vi "RT Driver VI.vi"(6 "Device Clock":string, 9 "Device Inputs FIFO":refnum<k33>, 10 "Device Outputs FIFO":refnum<k33>, 11 "Device Reference":T1 format="%.0x") -> ()   [LabVIEW 2018, in "CAN Gateway Engine.lvlib"]
uses:
  CAN Gateway Engine.lvlib
  <vilib>/NI Veristand/Custom Device API/Custom Device Item Ref.ctl
  <vilib>/Platform/TimedLoop/XDataNode/timing_clust.ctl
  <vilib>/Platform/TimedLoop/XDataNode/nitl_modes.ctl
  <vilib>/Platform/TimedLoop/XDataNode/wakeup.ctl
  <vilib>/platform/TimedLoop/XDataNode/XDataNode.xnode
  <vilib>/Platform/TimedLoop/XDataNode/XDNodeRunTimeDep.lvlib
  <vilib>/NI Veristand/Custom Device API/Custom Device API.lvlib
panel:
  in  "Initialization Status Notifier":refnum<notifier>
  in  "Status Notifier":refnum<notifier>
  # "Custom Device Template\nv1.0"
  # "Use this template as a starting point for creating a custom device code module. The input controls shown here are specially named controls that the system will use to provide the device loop with data. The controls are not required for the device loop to run. For instance, if the device doesn't produce any output data, then you don't need the Device Outputs FIFO control. If you do use these controls, however, they need to have these exact names to be functional."
  # "The optional status notifier element is used to notify the RT engine of the last state of the custom device, and to indicate the device has completed execution. If this control is not used, a default No Error value is returned to the system when the device finishes execution.\n\nNote: This error state is not checked until the system shuts down. Use an output status channel to send more immediate status values to the system."
  # "This optional input can be used to send the VeriStand Engine the final status of the custom device initalization process. If this control exists on the custom device front panel, the VeriStand Engine will wait for a status update before starting up. If the custom device reports an error, that will abort the execution of the current configuration in the VeriStand Engine.\n\nThis control can be deleted if the custom device does not need to send the initialization status update."
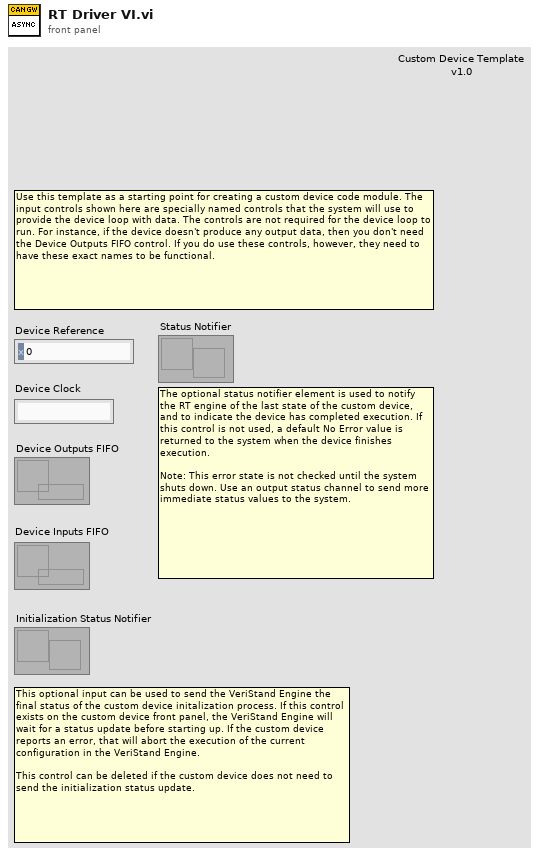
[diagram p1: front panel]
types:
  T1 = typedef "Custom Device API.lvlib/Custom Device Item Ref.ctl" = u64
  T2 = typedef "CAN Gateway Engine.lvlib/Runtime engine Data.ctl" = cluster{"Device Outputs FIFO":refnum<k33>, "Device Inputs FIFO":refnum<k33>, "CD In Size":i32, "CD Out Size":i32, "CD In Buf":dbl[], "CD Out Buf":dbl[], "Event Registration Refnum out":T3, "Specified Channel Ref List In":T1[], "Specified Channel Ref List Out":T1[], "Compiled Data":T4, "Read /write Sessions":cluster{"Network Read Session":refnum<k21>, "Network Write Session":refnum<k21>, "DUT Read Session":refnum<k21>, "DUT Write Session":refnum<k21>}}
  T3 = typedef "Custom Device API.lvlib/Custom Device Engine Event Ref.ctl" = refnum<event-registration>
  T4 = typedef "CAN Gateway Shared.lvlib/Compiled Data.ctl" = cluster{"HW Info Network Port":cluster{"CAN Port":string, "Baudrate":u64}, "HW Info DUT Port":cluster{"CAN Port":string, "Baudrate":u64}, "Corruption Info Network_DUT":T5, "Corruption Info DUT_Network":T5}
  T5 = typedef "CAN Gateway Shared.lvlib/Corruption Info.ctl" = cluster{"Corrupt IDs Array":u32[], "Frame Infos Array":T6[]}
  T6 = typedef "CAN Gateway Shared.lvlib/Frame.ctl" = cluster{"Disable Frame Channel Index":i32, "Has  CRC?":bool, "CRC start Bit":u32, "DLC corruption Channel Index":i32, "DLC Length  Corruption Index":i32, "CRC Index":i32, "Conversion Session":refnum<k21>, "CRC Signal":refnum<k21>, "Data Signal Array":T7[]}
  T7 = typedef "CAN Gateway Shared.lvlib/Signal_Data_Trigger.ctl" = cluster{"XNET Signal":refnum<k21>, "Data Idx":u32, "Trigger Idx":u32}
  T8 = typedef "XDNodeRunTimeDep.lvlib/timing_clust.ctl" = cluster{"Expected End [f-1]":u64, "Actual End [f-1]":u64, "Finished Late? [f-1]":bool, "Expected End [i-1]":u64, "Actual End [i-1]":u64, "Finished Late? [i-1]":bool, "Expected Start [i]":u64, "Actual Start [i]":u64, "Expected Start [f]":u64, "Actual Start [f]":u64, "Source Name":string, "Structure Name":string, "Period":i64, "Deadline":i64, "Offset":i64, "Start":i64, "Priority":i32, "Timeout":i32, "Mode":T9, "Wakeup Reason":T10, "Error":errorcluster, "Source Type":string, "Secondary Source Type":string, "Global End Time":u64, "Global Start Time":u64, "Frame Duration":u64, "Iteration Duration":u64, "Assigned CPU":i32, "I/O Scan Engine Mode":u32}
  T9 = typedef "XDNodeRunTimeDep.lvlib/nitl_modes.ctl" = enum32{"No Change", "Process missed periods, maintain original phase", "Discard missed periods, maintain original phase", "Process missed periods, ignore original phase", "Discard missed periods, ignore original phase"}
  T10 = typedef "XDNodeRunTimeDep.lvlib/wakeup.ctl" = enum32{"Normal", "Aborted", "Asynchronous wakeup", "Timing source error", "Timed loop error", "Timeout"}
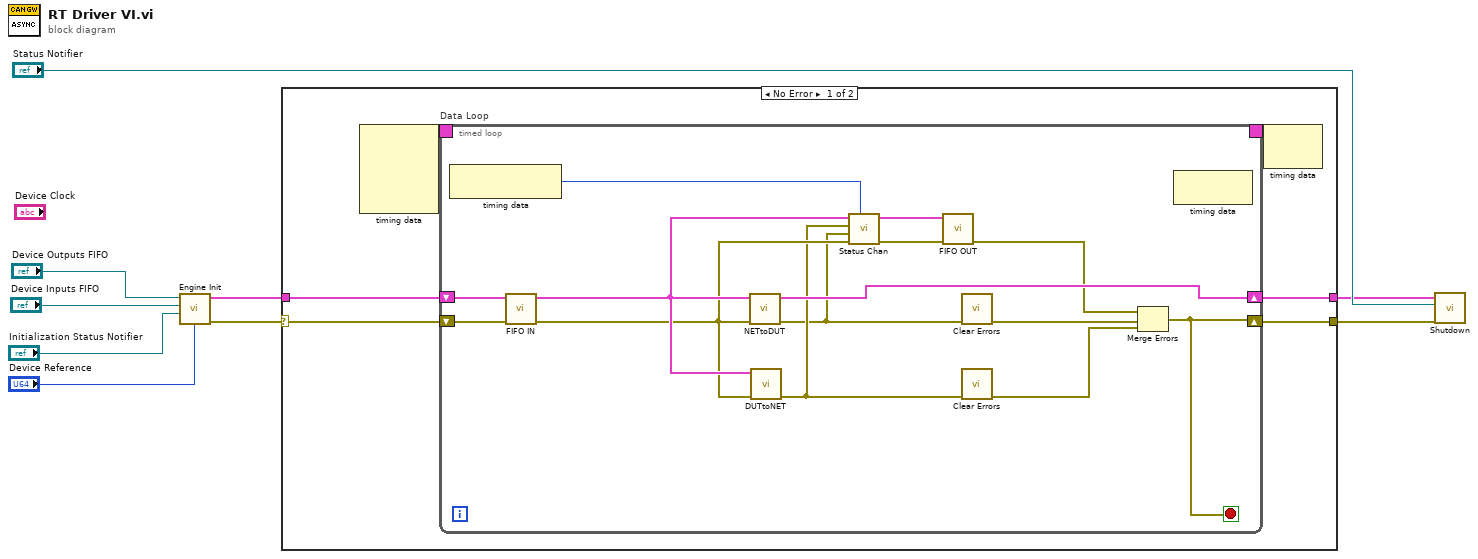
[diagram p0: block diagram]
diagram:
  n1 = call "Engine Init.vi"("Device Reference"="Device Reference", "Notifier in"="Initialization Status Notifier", "Device Inputs FIFO"="Device Inputs FIFO", "Device Outputs FIFO"="Device Outputs FIFO") -> ("error out"=w8:errorcluster, "Engine Run-Time Data Cluster"=w9:T2)  [unwired: 6 in]
  n2 = case shown="No Error" w8 {
    selector: w8 -> [w14 w36]
    tunnel: w9 -> [w11 w35]
    tunnel: [w15 w36] -> w3
    tunnel: [w10 w35] -> w1
    frame No Error {
      n3 = node-c288() -> (w13:T8)  [unwired: 4 in]
      n4 = timed-loop "Data Loop" {
        shift-right: [w23] -> w15
        shift-left: w14 -> [w29]
        shift-right: [w20] -> w10
        shift-left: w11 -> [w28]
        timing: w13 -> [_]
        timing-out: [_] -> w12
        stop <- w23 stop-if-true
        n5 = node-c288() -> (w18:i64)  [unwired: 1 in]
        n6 = call "FIFO IN.vi"("error in (no error)"=w29, "Engine Run-Time Data Cluster In"=w28) -> ("error out"=w26:errorcluster, "Engine Run-Time Data Cluster Out"=w27:T2)  [unwired: 8 in]
        n7 = call "NETtoDUT.vi"("error in (no error)"=w26, "Engine Run-Time Data Cluster In"=w27) -> ("error out"=w16:errorcluster, "Engine Run-Time Data Cluster Out"=w20:T2)  [unwired: 8 in]
        n8 = call "DUTtoNET.vi"("error in (no error)"=w26, "Engine Run-Time Data Cluster In"=w27) -> ("error out"=w17:errorcluster)  [unwired: 8 in, 1 out]
        n9 = call "Status Chan.vi"("Iteration Duration"=w18, "error in (no error)"=w26, "error Net to DUT"=w16, "error DUT to Net"=w17, "Engine Run-Time Data Cluster In"=w27) -> ("error out"=w25:errorcluster, "Engine Run-Time Data Cluster Out"=w24:T2)  [unwired: 5 in]
        n10 = call "FIFO OUT.vi"("error in (no error)"=w25, "Engine Run-Time Data Cluster In"=w24) -> ("error out"=w19:errorcluster)  [unwired: 8 in, 1 out]
        n11 = call <vilib>:"Clear Errors.vi"("error in (no error)"=w16) -> ("error out"=w22:errorcluster)  [unwired: 5 in, 1 out]
        n12 = call <vilib>:"Clear Errors.vi"("error in (no error)"=w17) -> ("error out"=w21:errorcluster)  [unwired: 5 in, 1 out]
        n13 = Merge Errors(w19, w22, w21) -> (w23:errorcluster)
        n14 = node-c288() -> ()  [unwired: 1 in, 1 out]
      }
      n15 = node-c288(w12) -> ()  [unwired: 1 out]
    }
    frame Error {
    }
  }
  n16 = call "Shutdown.vi"("error in (no error)"=w3, "Status Notifier"="Status Notifier", "Engine Run-Time Data Cluster In"=w1) -> ()  [unwired: 8 in, 1 out]
